vi "Assert Case and Method Status.vi"(8 "error in (no error)":errorcluster, 9 "Results":T1[](array[typedef]), 10 "Status":T2, 11 "Error Checking Test in":refnum<class "Error Checking Test.lvclass">) -> (0 "error out":errorcluster, 3 "Error Checking Test out":refnum<class "Error Checking Test.lvclass">)   [LabVIEW 2020, in "Error Checking Test.lvclass"]
uses:
  Error Checking Test.lvclass
  Result/Status.ctl
  Result/Result.ctl
  Result/Type.ctl
  C:/Program Files (x86)/National Instruments/LabVIEW 2020/vi.lib/Astemes/LUnit/Test Case.lvclass
  <vilib>/Astemes/LUnit/Test Case.lvclass/Test Case.ctl
  8297a807-aefa-40cb-be42-a36ff4bd44a4.vi
  <vilib>/Astemes/LUnit/Palette/Pass.vi
  <vilib>/Astemes/LUnit/Palette/Fail.vi
  <vilib>/Astemes/LUnit/Compare Variants.vi
  <vilib>/Astemes/LUnit/Describe Comparison.vi
  <vilib>/Astemes/LUnit/Set Assertion Type.vi
  <vilib>/Astemes/LUnit/Add test result.vi
  <vilib>/Astemes/LUnit/Variant to string.vi
  <vilib>/Astemes/LUnit/LUnit Record Assertion Result.vi
  <vilib>/Astemes/LUnit/LUnit Aggregate Assertion Results.vi
  <vilib>/Astemes/LUnit/Method Result/LUnit Merge Status.vi
  <vilib>/Astemes/LUnit/LUnit Concatenate result strings.vi
  <vilib>/Utility/Data Type/Get Type Information.vi
  <vilib>/Utility/LVClass/Get LV Class Name.vi
  Result/Result.lvlib
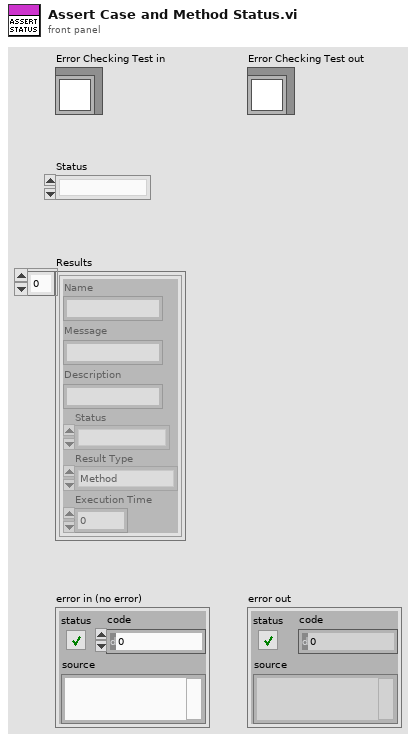
[diagram p1: front panel]
types:
  T1 = typedef "Result.lvlib/Result.ctl" = cluster{"Name":string, "Message":string, "Description":string, "Status":T2, "Result Type":T3, "Execution Time":dbl}
  T2 = typedef "Result.lvlib/Status.ctl" = enum16{"", "Passed", "Failed", "Error", "Skipped", "Setup Error", "Broken", "Teardown Error"}
  T3 = typedef "Result.lvlib/Type.ctl" = enum16{"Method", "Case", "Suite", "Pass", "Fail", "Skip", "Pass if", "Fail if", "Pass if Error", "Fail if Error", "Pass if Equal", "Fail if Equal"}
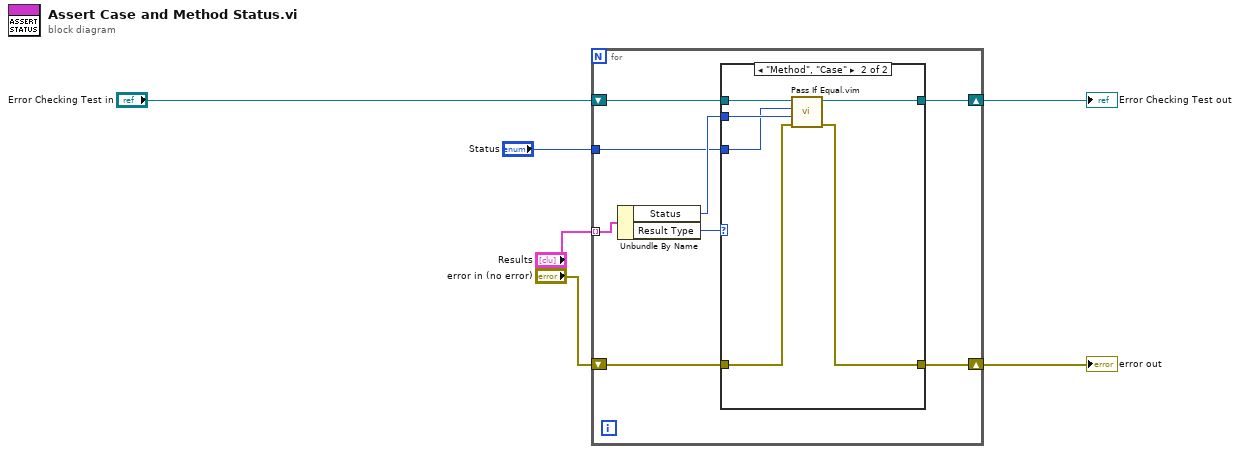
[diagram p0: block diagram]
diagram:
  n1 = for {
    tunnel: "Results" -> [w10] mode=indexing
    shift-right: [w13] -> w2
    shift-left: "Error Checking Test in" -> [w12]
    shift-right: [w14] -> w1
    shift-left: "error in (no error)" -> [w11]
    tunnel: "Status" -> [w7]
    n2 = Unbundle By Name(w10) -> ("Status"=w8:T2, "Result Type"=w9:T3)
    n3 = case shown="\"Method\", \"Case\"" w9 {
      tunnel: [w15 w22] -> w14
      tunnel: [w16 w21] -> w13
      tunnel: w12 -> [w16 w20]
      tunnel: w11 -> [w15 w19]
      tunnel: w8 -> [_ w18]
      tunnel: w7 -> [_ w17]
      frame Default {
      }
      frame "Method", "Case" {
        n4 = call "Pass If Equal.vim"("error in (no error)"=w19, "Actual"=w18, "Expected"=w17, "LUnit Test Case In"=w20) -> ("error out"=w22:errorcluster, "LUnit Test Case Out"=w21:refnum<class "Error Checking Test.lvclass">)  [unwired: 6 in]
      }
    }
  }
  "Error Checking Test out" <- w2
  "error out" <- w1
